vi "SetCommand.vi"(8 "error in (no error)":errorcluster, 10 "Command.lvclass":refnum<class "Command.lvclass">, 11 "Invoker in":refnum<class "Invoker.lvclass">) -> (0 "error out":errorcluster, 3 "Invoker out":refnum<class "Invoker.lvclass">)   [LabVIEW 2014, in "Invoker.lvclass"]
uses:
  Invoker.lvclass
  Command/Command.lvclass
  Invoker.lvclass/Invoker.ctl
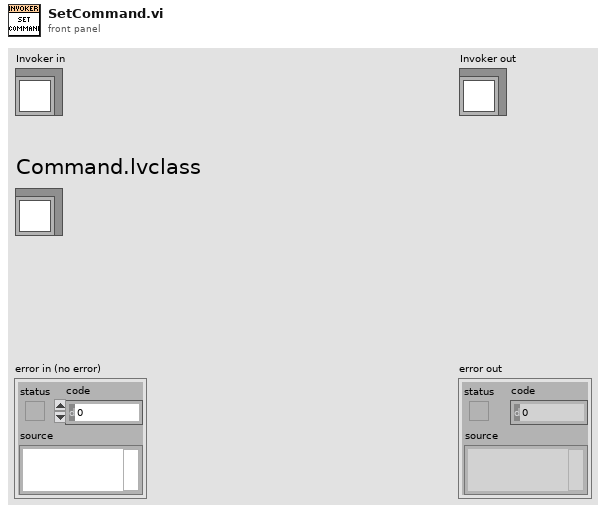
[diagram p1: front panel]
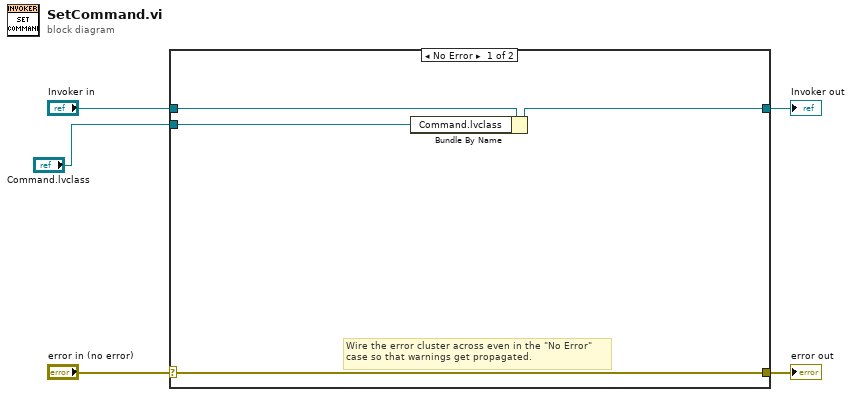
[diagram p0: block diagram]
diagram:
  n1 = case shown="No Error" "error in (no error)" {
    selector: "error in (no error)" -> [w8 w11]
    tunnel: [w8 w11] -> w4
    tunnel: [w7 w10] -> w2
    tunnel: "Invoker in" -> [w9 w10]
    tunnel: "Command.lvclass" -> [w6 _]
    frame No Error {
      # "Wire the error cluster across even in the \"No Error\"\ncase so that warnings get propagated."
      n2 = Bundle By Name(cluster=w9, "Command.lvclass"=w6) -> (w7:refnum<class "Invoker.lvclass">)
    }
    frame Error {
    }
  }
  "error out" <- w4
  "Invoker out" <- w2
